vi "Init DB-MySQL.vi"(8 "error in":errorcluster, 9 "Network Config":T2={"IP Address"="", "Port"=0, "Timeout ms"=500}, 10 "Authentication":T1, 11 "DB-MySQL in":refnum<class "DB-MySQL.lvclass">=refnum) -> (0 "error out":errorcluster, 3 "DB-MySQL out":refnum<class "DB-MySQL.lvclass">)   [LabVIEW 2014, in "hse-db.lvlib" / "DB-MySQL.lvclass"]
uses:
  DB-MySQL.lvclass
  Network Config.ctl
  DB-MySQL.lvclass/DB-MySQL.ctl
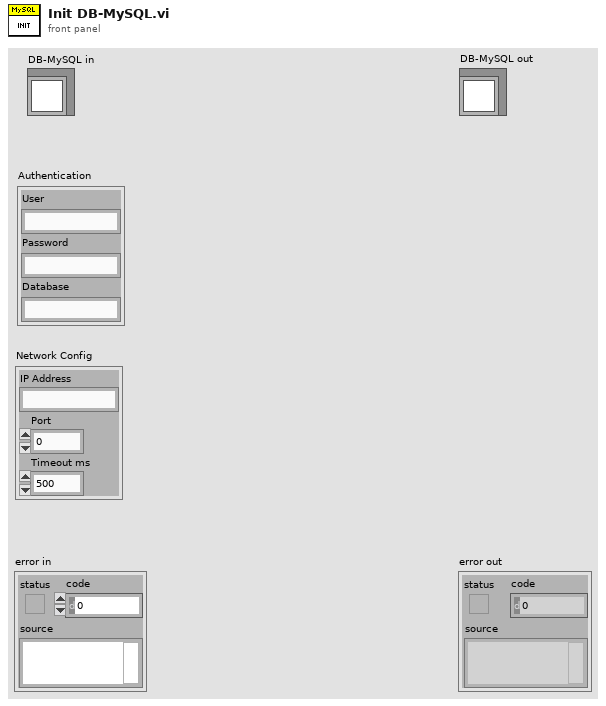
[diagram p1: front panel]
types:
  T1 = cluster{"User":string, "Password":string, "Database":string}
  T2 = typedef "hse-db.lvlib/DB-MySQL.lvclass/Network Config.ctl" = cluster{"IP Address":string, "Port":u16, "Timeout ms":i32}
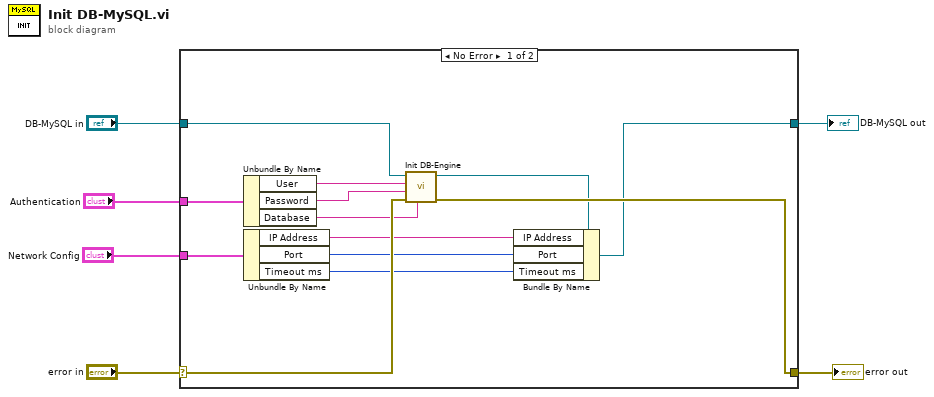
[diagram p0: block diagram]
diagram:
  n1 = case shown="No Error" "error in" {
    selector: "error in" -> [w19 w21]
    tunnel: [w18 w21] -> w5
    tunnel: [w17 w20] -> w4
    tunnel: "DB-MySQL in" -> [w16 w20]
    tunnel: "Network Config" -> [w11 _]
    tunnel: "Authentication" -> [w7 _]
    frame No Error {
      n2 = Unbundle By Name(w7) -> ("User"=w14:string, "Password"=w13:string, "Database"=w12:string)
      n3 = Unbundle By Name(w11) -> ("IP Address"=w10:string, "Port"=w9:u16, "Timeout ms"=w8:i32)
      n4 = call-dynamic "Init DB-Engine.vi"("Database"=w12, "error in"=w19, "Password"=w13, "User"=w14, "DB-Engine in"=w16) -> ("error out"=w18:errorcluster, "DB-Engine out"=w15:refnum<class "DB-MySQL.lvclass">)  [unwired: 5 in]
      n5 = Bundle By Name(cluster=w15, "IP Address"=w10, "Port"=w9, "Timeout ms"=w8) -> (w17:refnum<class "DB-MySQL.lvclass">)
    }
    frame Error {
    }
  }
  "error out" <- w5
  "DB-MySQL out" <- w4
